vi "Encoder_RefNum Registry Get.vi"(2 "error in (no error)":errorcluster, 3 "refnum name":string="RobotDrive") -> (0 "error out":errorcluster, 1 "RobotEncoderRef Out":T5)   [LabVIEW 2013]
uses:
  <vilib>/Rock Robotics/WPI/Encoder/WPI_EncoderDevRef.ctl
  <vilib>/Rock Robotics/SystemInterfaces/Encoder/FPGA_EncoderIdx.ctl
  <vilib>/Rock Robotics/SystemInterfaces/Counter/FPGA_CounterCtrSystemIndex.ctl
  <vilib>/Rock Robotics/WPI/Encoder/WPI_EncoderType.ctl
  <vilib>/Rock Robotics/WPI/Utilities/Refnum Registry Operation.ctl
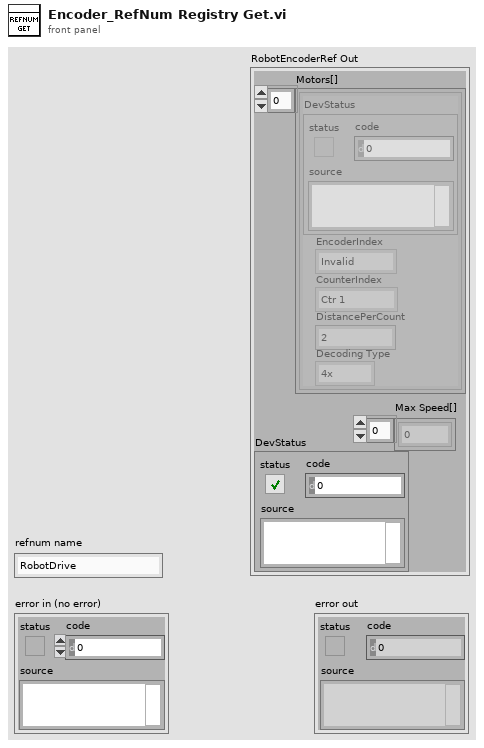
[diagram p1: front panel]
types:
  T1 = typedef "WPI_EncoderDevRef.ctl" = cluster{"DevStatus":errorcluster, "EncoderIndex":T2, "CounterIndex":T3, "DistancePerCount":dbl, "Decoding Type":T4}
  T2 = typedef "FPGA_EncoderIdx.ctl" = enum8{"Enc 0", "Enc 1", "Enc 2", "Enc 3", "Invalid"}
  T3 = typedef "FPGA_CounterCtrSystemIndex.ctl" = enum8{"Ctr 0", "Ctr 1", "Ctr 2", "Ctr 3", "Ctr 4", "Ctr 5", "Ctr 6", "Ctr 7", "Invalid"}
  T4 = typedef "WPI_EncoderType.ctl" = enum16{"1x", "2x", "4x"}
  T5 = cluster{"Motors[]":T1[], "DevStatus":errorcluster, "Max Speed[]":dbl[]}
  T6 = typedef "Refnum Registry Operation.ctl" = enum16{"set", "get", "delete", "get all names", "read name"}
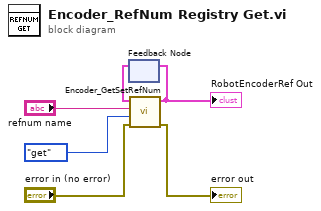
[diagram p0: block diagram]
diagram:
  n1 = feedback #1() -> (w6:T5)  [unwired: 1 in]
  n2 = call "Encoder_GetSetRefNum.vi"("error in (no error)"="error in (no error)", "menu"=Refnum_Registry_Operation."get", "refnum name"="refnum name", "RobotEncoderRef"=w6) -> ("error out"=→"error out":errorcluster, "RobotEncoderRef Out"=w1:T5)  [unwired: 5 in, 1 out]
  "RobotEncoderRef Out" <- w1
  n3 = feedback-in #1(w1) -> ()
